vi "StrainDAQ_B.vi"() -> (15 "Strain Array":i32[](array[numeric]), 20 "element_1":i32, 21 "element_2":i32, 22 "element_3":i32, 23 "element_4":i32, 24 "element_5":i32, 25 "element_6":i32, 26 "element_7":i32, 27 "element_8":i32)   [LabVIEW 2013]
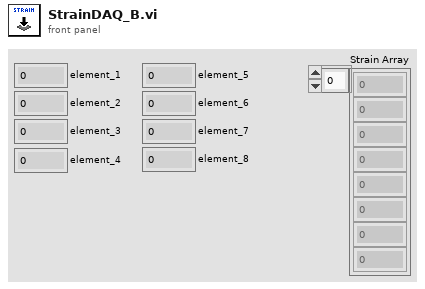
[diagram p1: front panel]
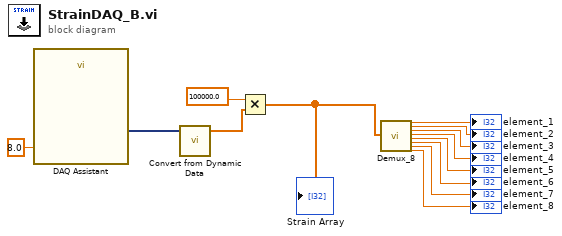
[diagram p0: block diagram]
diagram:
  n1 = call "DAQ Assistant"("timeout (s)"=8.0) -> ("data"=w13:dynamicdata)  [unwired: 16 in, 2 out]
  n2 = call "Convert from Dynamic Data"("Dynamic Data Type"=w13) -> ("Array"=w10:dbl[])  [unwired: 3 in]
  n3 = Multiply(x=100000.0, y=w10) -> (x*y=w9:dbl[])
  "Strain Array" <- w9
  n4 = call "Demux_8.vi"("Data_Array"=w9) -> ("element_1"=→"element_1":dbl, "element_2"=→"element_2":dbl, "element_3"=→"element_3":dbl, "element_4"=→"element_4":dbl, "element_5"=→"element_5":dbl, "element_6"=→"element_6":dbl, "element_7"=→"element_7":dbl, "element_8"=→"element_8":dbl)  [unwired: 19 in]
